vi "symbol update.vi"(1 "from index":i32, 2 "current":i32, 3 "total row":i64) -> (0 "symbol":i32[](array[numeric]))   [LabVIEW 2025]
doc: "Author: Scott Hannahs <sth@magnet.fsu.edu>\n\nThis software is licensed for use under the “MIT License\"\nCopyright (c) 2025 Scott Hannahs, sth@sth@magnet.sthnet.net\n\nPermission is hereby granted, free of charge, to any person obtaining a copy of this software and associated documentation files (the \"Software\"), to deal in the Software without restriction, including without limitation the rights to use, copy, modify, merge, publish, distribute, sublicense, and/or sell copies of the Software, and to permit persons to whom the Software is furnished to do so, subject to the following conditions: The above copyright notice and this permission notice shall be included in all copies or substantial portions of the Software.\n\nTHE SOFTWARE IS PROVIDED \"AS IS\", WITHOUT WARRANTY OF ANY KIND, EXPRESS OR IMPLIED, INCLUDING BUT NOT LIMITED TO THE WARRANTIES OF MERCHANTABILITY, FITNESS FOR A PARTICULAR PURPOSE AND NONINFRINGEMENT. IN NO EVENT SHALL THE AUTHORS OR COPYRIGHT HOLDERS BE LIABLE FOR ANY CLAIM, DAMAGES OR OTHER LIABILITY, WHETHER IN AN ACTION OF CONTRACT, TORT OR OTHERWISE, ARISING FROM, OUT OF OR IN CONNECTION WITH THE SOFTWARE OR THE USE OR OTHER DEALINGS IN THE SOFTWARE."
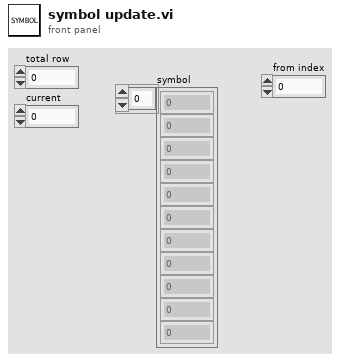
[diagram p1: front panel]
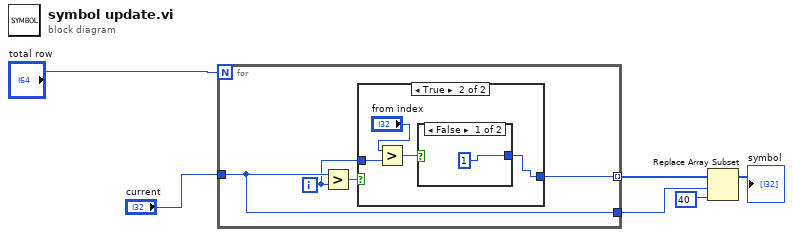
[diagram p0: block diagram]
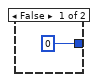
[diagram p2: hidden frame]
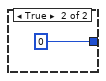
[diagram p3: hidden frame]
diagram:
  n1 = for {
    N: "total row" -> [_]
    tunnel: [w10] -> w6 mode=indexing
    tunnel: "current" -> [w8]
    tunnel: [w8] -> w1
    i -> [w7]
    n2 = Greater?(x=w8, y=w7) -> (0:w9:bool)
    n3 = case shown="True" w9 {
      tunnel: [0 w12] -> w10
      tunnel: w7 -> [_ w13]
      frame False {
      }
      frame True {
        n4 = Greater?(x="from index", y=w13) -> (0:w15:bool)
        n5 = case shown="False" w15 {
          tunnel: [1 0] -> w12
          frame False {
          }
          frame True {
          }
        }
      }
    }
  }
  n6 = Replace Array Subset(array=w6, new element=40 ("new element/subarray"), index=w1) -> (→"symbol":i32[])
